vi "Cal RHS (VIRef).vi"(8 "error in (no error)":errorcluster, 10 "RHS in":variant, 11 "Domain_Evolut_2D_Rect in":refnum<class "NI_Domain_Evolut_2D_Rect.lvclass">) -> (0 "error out":errorcluster, 2 "RHS out":variant, 3 "Domain_Evolut_2D_Rect out":refnum<class "NI_Domain_Evolut_2D_Rect.lvclass">)   [LabVIEW 2020, in "NI_PDE.lvlib" / "NI_Domain_Evolut_2D_Rect.lvclass"]
uses:
  <vilib>/gmath/pde.llb/DomainClass/Domain_Evolut_2D_Rect/NI_Domain_Evolut_2D_Rect.lvclass
  <vilib>/gmath/pde.llb/RHSClass/RHS_3D_VIRef/RHS Data.ctl
  <vilib>/gmath/pde.llb/DomainClass/Domain_Evolut_2D_Rect/NI_Domain_Evolut_2D_Rect.lvclass/NI_Domain_Evolut_2D_Rect.ctl
  <vilib>/Analysis/1siggen.llb/Ramp Pattern by Samples.vi
  <vilib>/gmath/pde.llb/RHSClass/RHS_3D_VIRef/NI_RHS_3D_VIRef.lvclass
  <vilib>/gmath/NI_PDE.lvlib
  <vilib>/Analysis/NI_AALBase.lvlib
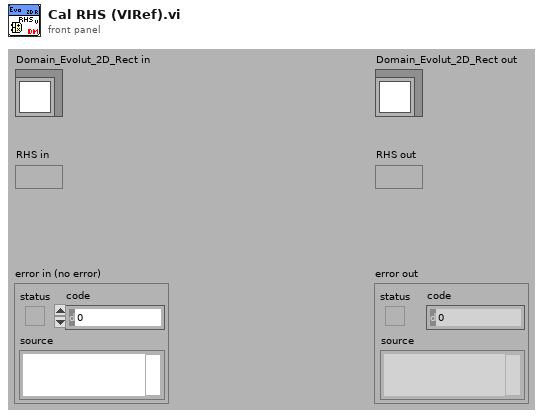
[diagram p1: front panel]
types:
  T1 = typedef "NI_PDE.lvlib/NI_RHS_3D_VIRef.lvclass/RHS Data.ctl" = cluster{"F":refnum<vi>, "data":variant}
  T2 = cluster{"initial t":dbl, "final t":dbl, "# of t-points":i32}
  T3 = cluster{"start x":dbl, "end x":dbl, "# of x-points":i32}
  T4 = cluster{"start y":dbl, "end y":dbl, "# of y-points":i32}
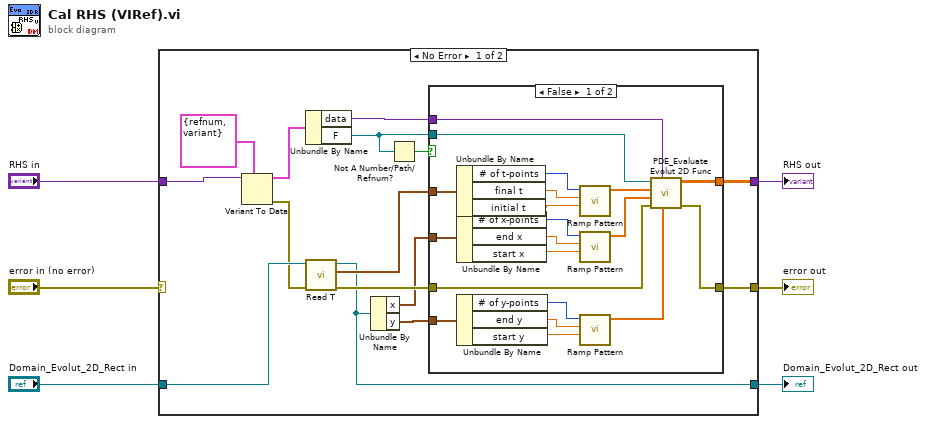
[diagram p0: block diagram]
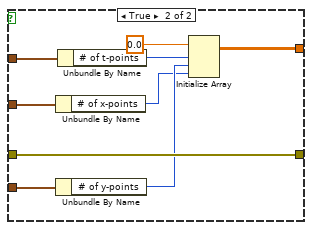
[diagram p2: hidden frame]
diagram:
  n1 = case shown="No Error" "error in (no error)" {
    selector: "error in (no error)" -> [_ w53]
    tunnel: "Domain_Evolut_2D_Rect in" -> [w14 w52]
    tunnel: [w9 w52] -> w6
    tunnel: [w10 w53] -> w5
    tunnel: [w11 w51] -> w2
    tunnel: "RHS in" -> [w21 w51]
    frame No Error {
      n2 = Variant To Data(type=T1 {"F"=refnum, "data"=variant} ("RHS data"), Variant=w21) -> (data=w12:T1, error out=w13:errorcluster)  [unwired: 1 in]
      n3 = Unbundle By Name(w12) -> ("data"=w17:variant, "F"=w16:refnum<vi>)
      n4 = call-dynamic "Read T.vi"("error in (no error)"=w13, "Domain_Evolut.lvclass in"=w14) -> ("error out"=w18:errorcluster, "t"=w19:T2, "Domain_Evolut.lvclass out"=w9:refnum<class "NI_Domain_Evolut_2D_Rect.lvclass">)  [unwired: 7 out]
      n5 = Unbundle By Name(w9) -> ("x"=w8:T3, "y"=w7:T4)
      n6 = Not A Number/Path/Refnum?(number/path/refnum=w16) -> (NaN/Path/Refnum?=w15:bool)
      n7 = case shown="False" w15 {
        tunnel: [w31 w50] -> w11
        tunnel: w19 -> [w41 w49]
        tunnel: w8 -> [w34 w48]
        tunnel: w16 -> [w33 _]
        tunnel: w17 -> [w32 _]
        tunnel: w18 -> [w30 w46]
        tunnel: [w29 w46] -> w10
        tunnel: w7 -> [w24 w44]
        frame False {
          n8 = Unbundle By Name(w41) -> ("# of t-points"=w39:i32, "final t"=w38:dbl, "initial t"=w40:dbl)
          n9 = Unbundle By Name(w34) -> ("# of x-points"=w36:i32, "end x"=w37:dbl, "start x"=w35:dbl)
          n10 = Unbundle By Name(w24) -> ("# of y-points"=w22:i32, "end y"=w25:dbl, "start y"=w26:dbl)
          n11 = call-poly <vilib>:"Ramp Pattern.vi"("start"=w40, "end"=w38, "samples"=w39) -> ("Ramp Pattern"=w28:dbl[])  [unwired: 7 in, 1 out]
          n12 = call-poly <vilib>:"Ramp Pattern.vi"("start"=w35, "end"=w37, "samples"=w36) -> ("Ramp Pattern"=w27:dbl[])  [unwired: 7 in, 1 out]
          n13 = call-poly <vilib>:"Ramp Pattern.vi"("start"=w26, "end"=w25, "samples"=w22) -> ("Ramp Pattern"=w23:dbl[])  [unwired: 7 in, 1 out]
          n14 = call <vilib>:"PDE_Evaluate Evolut 2D Func.vi"("Y"=w23, "data"=w32, "error in (no error)"=w30, "X"=w27, "T"=w28, "VIRef"=w33) -> ("error out"=w29:errorcluster, "F(t, x, y)"=w31:dbl[][][])  [unwired: 4 out]
        }
        frame True {
          n15 = Unbundle By Name(w48) -> ("# of x-points"=w42:i32)
          n16 = Unbundle By Name(w44) -> ("# of y-points"=w43:i32)
          n17 = Unbundle By Name(w49) -> ("# of t-points"=w45:i32)
          n18 = Initialize Array(0.0 ("element"), w45, w43, w42) -> (w50:dbl[][][])
        }
      }
    }
    frame Error {
    }
  }
  "Domain_Evolut_2D_Rect out" <- w6
  "error out" <- w5
  "RHS out" <- w2
